vi "get_value.vi"(8 "error in (no error)":errorcluster, 10 "channel":dbl, 11 "Pfeiffer MultiGauge TPG256 in":refnum<class "Pfeiffer MultiGauge TPG256.lvclass">) -> (0 "error out":errorcluster, 2 "value":string, 3 "Pfeiffer MultiGauge TPG256 out":refnum<class "Pfeiffer MultiGauge TPG256.lvclass">)   [LabVIEW 2018, in "Pfeiffer MultiGauge TPG256.lvclass"]
doc: "the vi reads the value (pressure, temp etc etc) from the instrument"
uses:
  Pfeiffer MultiGauge TPG256.lvclass
  instrument.lvclass
  Drivers/Pfeiffer_MaxiGauge/Maxi Gauge.lvlib
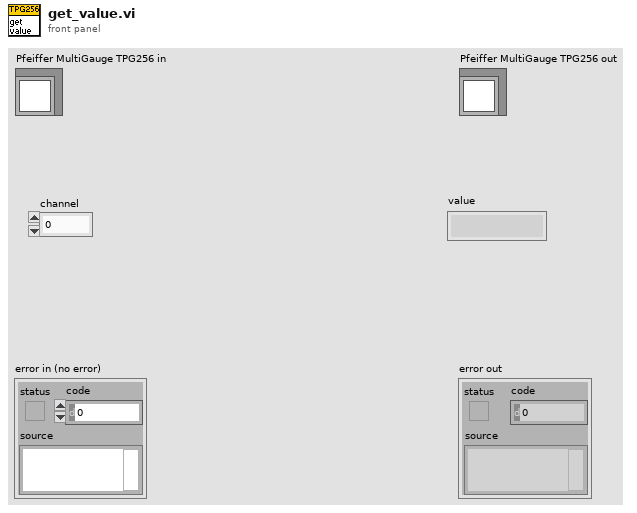
[diagram p1: front panel]
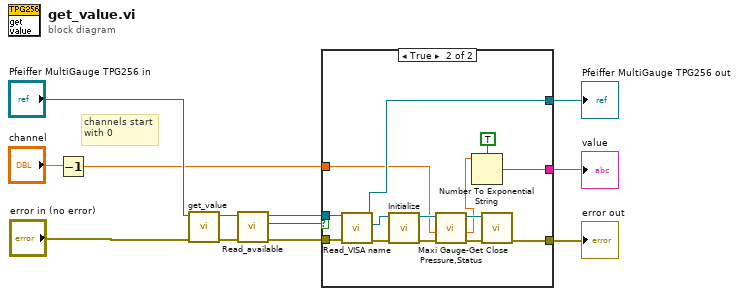
[diagram p0: block diagram]
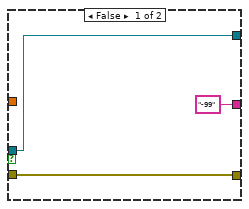
[diagram p2: hidden frame]
diagram:
  # "channels start\nwith 0"
  n1 = Decrement(x="channel") -> (x-1=w7:dbl)
  n2 = call-parent "get_value.vi"("error in (no error)"="error in (no error)", "instrument in"="Pfeiffer MultiGauge TPG256 in") -> ("error out"=w5:errorcluster, "instrument out"=w6:refnum<class "Pfeiffer MultiGauge TPG256.lvclass">)  [unwired: 7 in, 1 out]
  n3 = call-dynamic "Read_available.vi"("error in (no error)"=w5, "instrument in"=w6) -> ("error out"=w3:errorcluster, "available?"=w1:bool, "instrument out"=w4:refnum<class "Pfeiffer MultiGauge TPG256.lvclass">)  [unwired: 7 in]
  n4 = case shown="True" w1 {
    tunnel: [w15 w23] -> w10
    tunnel: ["-99" w22] -> w9
    tunnel: w7 -> [_ w20]
    tunnel: w4 -> [w15 w19]
    tunnel: w3 -> [w14 w18]
    tunnel: [w14 w17] -> w2
    frame False {
    }
    frame True {
      n5 = call-dynamic "Read_VISA name.vi"("error in (no error)"=w18, "instrument in"=w19) -> ("error out"=w28:errorcluster, "VISA resource name"=w29:refnum<visa-resource-name>, "instrument out"=w23:refnum<class "Pfeiffer MultiGauge TPG256.lvclass">)  [unwired: 7 in]
      n6 = call "Initialize.vi"("error in (no error)"=w28, "input refnum"=w29) -> ("error out"=w26:errorcluster, "VISA resource out"=w27:refnum<visa-resource-name>)  [unwired: 8 in]
      n7 = call "Maxi Gauge-Get Pressure,Status.vi"("Fehler (Eingang, kein Fehler)"=w26, "Sensor Nr.:"=w20, "VISA-Ressource in"=w27) -> ("Fehler (Ausgang)"=w24:errorcluster, "Pressure"=w21:dbl, "VISA-Ressource out"=w25:refnum<visa-resource-name>)  [unwired: 5 in, 1 out]
      n8 = Number To Exponential String(number=w21, 1:TRUE ("use system decimal point (T)")) -> (E-format string=w22:string)  [unwired: 2 in]
      n9 = call "Close.vi"("error in (no error)"=w24, "VISA resource name"=w25) -> ("error out"=w17:errorcluster)  [unwired: 9 in]
    }
  }
  "error out" <- w2
  "Pfeiffer MultiGauge TPG256 out" <- w10
  "value" <- w9
